vi "FileOperationRead.vi"() -> ()   [LabVIEW 2019]
panel:
  in  "stop":bool
  in  "Clear":bool
  in  "Read":bool
  out "text":string
  in  "?":path
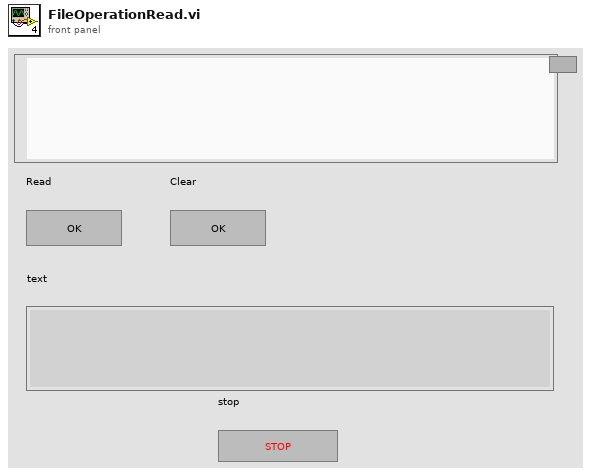
[diagram p1: front panel]
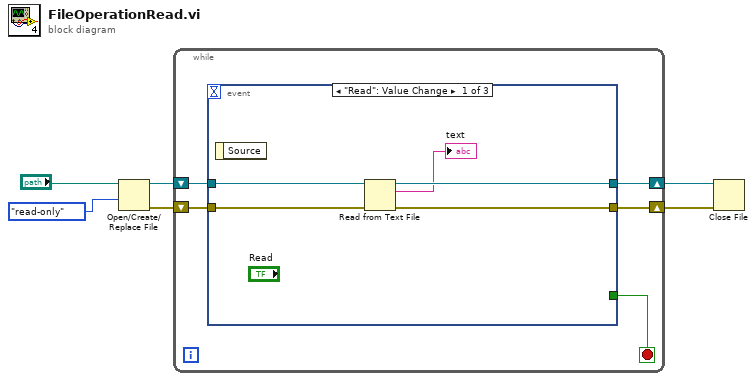
[diagram p0: block diagram]
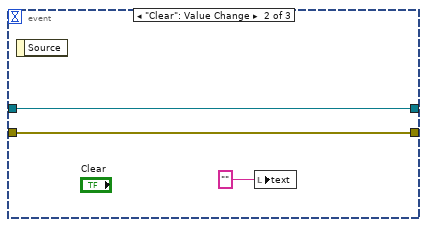
[diagram p2: hidden frame]
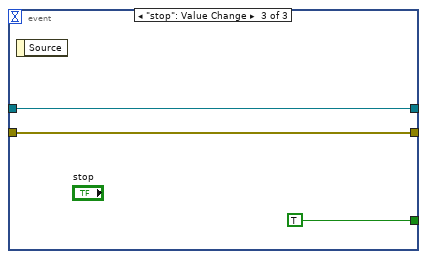
[diagram p3: hidden frame]
diagram:
  n1 = Open/Create/Replace File(file path (use dialog)="?", access (0:read/write)=enum16{"read/write", "read-only", "write-only"}."read-only") -> (refnum out=w4:refnum<file>, error out=w5:errorcluster)  [unwired: 4 in, 1 out]
  n2 = while {
    shift-right: [w8] -> w2
    shift-left: w5 -> [w11]
    shift-right: [w9] -> w3
    shift-left: w4 -> [w10]
    stop <- w7 stop-if-true
    n3 = event shown="[0] \"Read\": Value Change" {
      selector: _ -> [_ _ _]
      dyn-events: _ -> [_ _ _]
      timeout: _ -> [_ _ _]
      tunnel: w11 -> [w16 w18 w20]
      tunnel: w10 -> [w15 w19 w21]
      tunnel: [w14 w19 w21] -> w9
      tunnel: [w13 w18 w20] -> w8
      tunnel: [_ _ TRUE] -> w7
      event "Read": Value Change {
        n4 = event-data() -> ()  [unwired: 1 in, 1 out]
        n5 = Read from Text File(file (use dialog)=w15, error in=w16) -> (refnum out=w14:refnum<file>, text=→"text":string, error out=w13:errorcluster)  [unwired: 2 in, 1 out]
      }
      event "Clear": Value Change {
        n6 = event-data() -> ()  [unwired: 1 in, 1 out]
        n7 = local write "text"("") -> ()
      }
      event "stop": Value Change {
        n8 = event-data() -> ()  [unwired: 1 in, 1 out]
      }
    }
  }
  n9 = Close File(refnum=w3, error in=w2) -> ()  [unwired: 2 out]
